vi "Configure Response.vi"   [LabVIEW 2018, in "Instrument Addon Scripting API.lvlib"]
doc: "Configures the input response with the specified settings.\n \nIf you want to use Linked Channels with the Response Format string, ensure the Channel Refnums used in the Linked Channels parameter already exist before calling this SubVI. \n\nAn error will occur in the following situations: \n- The Response Format string contains duplicate Variable Names. \n- The number of variables in the Response Format string differ from the number of Linked Channels.\n- The Variable Names in the Response Format string differ from the Variable Names used in the Linked Channels parameter."
uses:
  Instrument Addon Scripting API.lvlib
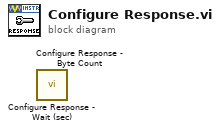
[diagram p0: block diagram]
diagram:
  n1 = call "Configure Response - Wait (sec).vi"() -> ()  [unwired: 10 in, 2 out]
  n2 = call "Configure Response - Byte Count.vi"() -> ()  [unwired: 10 in, 2 out]
